vi "SS_3phase_Sig_Gen.vi"(8 "error in (no error)":errorcluster, 11 "SSTestInfoCluster":T1={"Signal Information"=[{"Af"=1.0, "Phf"=0.0, "dc"=0.0, "Ah"=0.0, "phh"=0.0}, {"Af"=1.0, "Phf"=-120.0, "dc"=0.0, "Ah"=0.0, "phh"=-120.0}, {"Af"=1.0, "Phf"=120.0, "dc"=0.0, "Ah"=0.0, "phh"=120.0}, {"Af"=0.5, "Phf"=0.0, "dc"=0.0, "Ah"=0.0, "phh"=0.0}, {"Af"=0.5, "Phf"=-120.0, "dc"=0.0, "Ah"=0.0, "phh"=-120.0}, {"Af"=0.5, "Phf"=120.0, "dc"=0.0, "Ah"=0.0, "phh"=120.0}], "Test InfoSS"={"Fc"=60.0, "Interharmonic"=30.0, "Gen rate"=100000.0, "GenSampls"=1000000, "SmplIntvl s"=5.0, "sampl rate"=48000.0, "sample mode"=10178, "NI Cycles"=3.0, "Delay"=5.0, "Fit Harmonics"=1, "F0"=1.0, "Fs"=1.0}} {"Test InfoSS"."sample mode" items=["Finite Samples"=10178, "Continuous Samples"=10123, "Hardware Timed Single Point"=12522]}) -> (0 "error out":errorcluster, 3 "Generated waveforms":waveform(dbl)[](array[waveform])=[{"t0"=timestamp(0 s since 1904-01-01), "dt"=1.0, "Y"=array[5000 elements]}, {"t0"=timestamp(0 s since 1904-01-01), "dt"=1.0, "Y"=array[5000 elements]}, {"t0"=timestamp(0 s since 1904-01-01), "dt"=1.0, "Y"=array[5000 elements]}, {"t0"=timestamp(0 s since 1904-01-01), "dt"=1.0, "Y"=array[5000 elements]}, {"t0"=timestamp(0 s since 1904-01-01), "dt"=1.0, "Y"=array[5000 elements]}, {"t0"=timestamp(0 s since 1904-01-01), "dt"=1.0, "Y"=array[5000 elements]}], 4 "DataSamples":dbl[][](array[numeric]))   [LabVIEW 2014]
uses:
  TypeDefs/SSTestInfoCluster.ctl
  TypeDefs/SignalInfo.ctl
  TypeDefs/Test InfoSS.ctl
panel:
  out "Waveform Chart":waveform(dbl)[](graph)=[{"t0"=timestamp(0 s since 1904-01-01), "dt"=1.0, "Y"=array[5000 elements]}, {"t0"=timestamp(0 s since 1904-01-01), "dt"=1.0, "Y"=array[5000 elements]}, {"t0"=timestamp(0 s since 1904-01-01), "dt"=1.0, "Y"=array[5000 elements]}, {"t0"=timestamp(0 s since 1904-01-01), "dt"=1.0, "Y"=array[5000 elements]}, {"t0"=timestamp(0 s since 1904-01-01), "dt"=1.0, "Y"=array[5000 elements]}, {"t0"=timestamp(0 s since 1904-01-01), "dt"=1.0, "Y"=array[5000 elements]}]
  # "Af*cos(2*Pi*Fc*t+Phf) + Ah*cos(2*Pi*Fh*t+Phh) + dc"
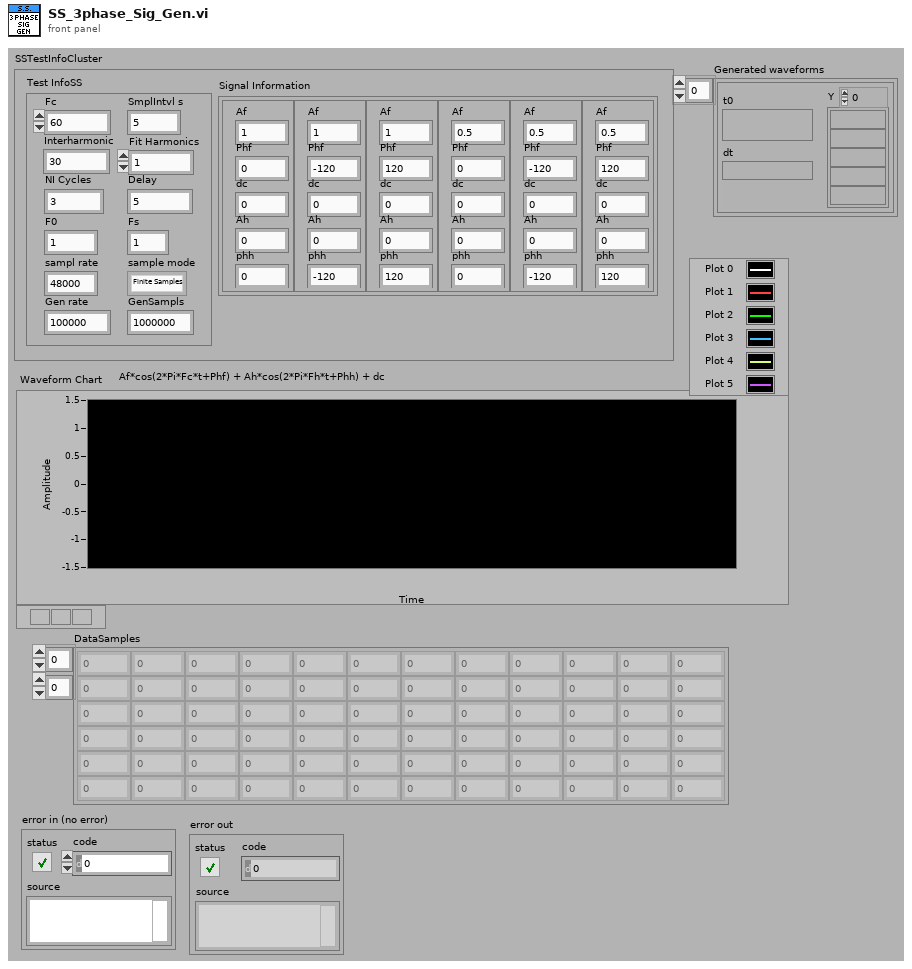
[diagram p1: front panel]
types:
  T1 = typedef "SSTestInfoCluster.ctl" = cluster{"Signal Information":T2, "Test InfoSS":T3}
  T2 = typedef "SignalInfo.ctl" = cluster{"Af":dbl, "Phf":dbl, "dc":dbl, "Ah":dbl, "phh":dbl}[]
  T3 = typedef "Test InfoSS.ctl" = cluster{"Fc":dbl, "Interharmonic":dbl, "Gen rate":dbl, "GenSampls":i32, "SmplIntvl s":dbl, "sampl rate":dbl, "sample mode":i32, "NI Cycles":dbl, "Delay":dbl, "Fit Harmonics":i32, "F0":dbl, "Fs":dbl}
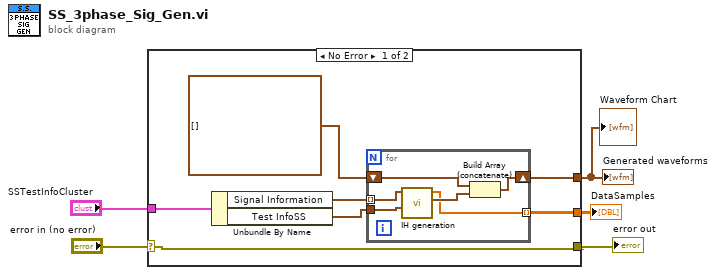
[diagram p0: block diagram]
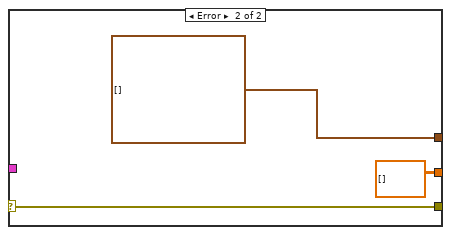
[diagram p2: hidden frame]
diagram:
  n1 = case shown="No Error" "error in (no error)" {
    selector: "error in (no error)" -> [w7 w21]
    tunnel: [w11 waveform(dbl)[] []] -> w2
    tunnel: "SSTestInfoCluster" -> [w10 _]
    tunnel: [w7 w21] -> w3
    tunnel: [w6 dbl[][] [] ("DataSamples")] -> w1
    frame No Error {
      n2 = Unbundle By Name(w10) -> ("Signal Information"=w9:T2, "Test InfoSS"=w8:T3)
      n3 = for {
        tunnel: w9 -> [w15] mode=indexing
        shift-right: [w17] -> w11
        shift-left: waveform(dbl)[] [] -> [w16]
        tunnel: w8 -> [w14]
        tunnel: [w13] -> w6 mode=indexing
        n4 = call "IH generation.vi"("Test InfoSS"=w14, "Signal Info"=w15) -> ("Single Phase"=w18:waveform(dbl), "DataSamples"=w13:dbl[])  [unwired: 8 in]
        n5 = Build Array (concatenate)(w16, w18) -> (w17:waveform(dbl)[])
      }
    }
    frame Error {
    }
  }
  "Generated waveforms" <- w2
  "error out" <- w3
  "Waveform Chart" <- w2
  "DataSamples" <- w1
